vi "Decode Return Codes.vi"(10 "Return Codes":u8[](array[numeric]) format="%08b") -> (1 "Invalid Code?":bool, 2 "Subscription Success":T1[](array[typedef]))   [LabVIEW 2013, in "SUBACK.lvclass"]
uses:
  SUBACK.lvclass
  Subscription Success Code.ctl
  ControlPacket/QualityOfService -- enum.ctl
  ControlPacket/ControlPacket.lvclass
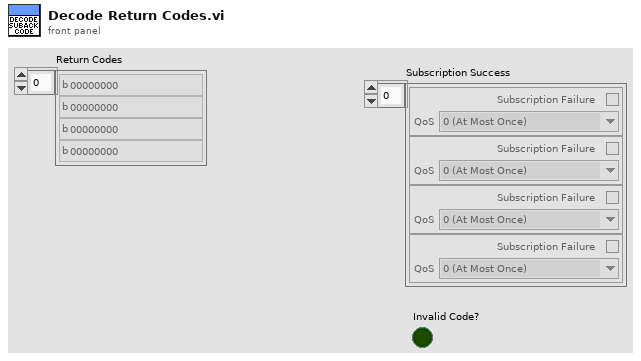
[diagram p1: front panel]
types:
  T1 = typedef "SUBACK.lvclass/Subscription Success Code.ctl" = cluster{"Subscription Failure":bool, "QoS":T2}
  T2 = typedef "ControlPacket.lvclass/QualityOfService -- enum.ctl" = enum16{"0 (At Most Once)", "1 (At Least Once)", "2 (Exactly Once)"}
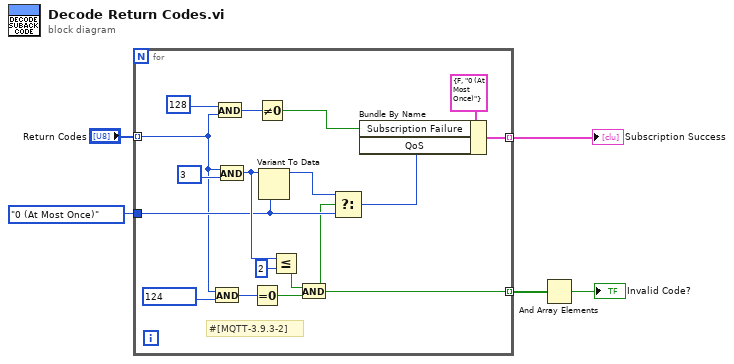
[diagram p0: block diagram]
diagram:
  n1 = for {
    tunnel: "Return Codes" -> [w11] mode=indexing
    tunnel: [w21] -> w4 mode=indexing
    tunnel: [w6] -> w3 mode=indexing
    tunnel: QualityOfService_--_enum."0 (At Most Once)" ("QoS") -> [w15]
    # "#[MQTT-3.9.3-2]"
    n2 = And(x=w11, y=u8 124) -> (x .and. y?=w10:u8)
    n3 = And(x=u8 128 ("y"), y=w11) -> (x .and. y?=w19:u8)
    n4 = And(x=w11, y=u8 3) -> (x .and. y?=w16:u8)
    n5 = Equal To 0?(x=w10) -> (x = 0?=w7:bool)
    n6 = Not Equal To 0?(x=w19) -> (x != 0?=w18:bool)
    n7 = Variant To Data(type=w15, Variant=w16) -> (data=w14:T2)  [unwired: 1 in, 1 out]
    n8 = Less Or Equal?(x=w16, y=u8 2) -> (x <= y?=w8:bool)
    n9 = And(x=w8, y=w7) -> (x .and. y?=w6:bool)
    n10 = Select(t=w14, s=w6, f=w15) -> (s? t:f=w13:T2)
    n11 = Bundle By Name(cluster=T1 {"Subscription Failure"=FALSE, "QoS"=enum."0 (At Most Once)"} ("Topic Subscription"), "Subscription Failure"=w18, "QoS"=w13) -> (w21:T1)
  }
  "Subscription Success" <- w4
  n12 = And Array Elements(Boolean array=w3) -> (logical AND=→"Invalid Code?":bool)
